vi "Pockels Cal-Interpolate or Condense.vi"(9 "Processing Type (Interpolate)":T1, 11 "Pockels Cal table":string[][](array[string])=[["0", "0", "0", "0"], ["0.1", "", "", ""], ["0.2", "", "6.86", ""], ["0.3", "", "", ""], ["0.4", "37.1", "25.97", "37.1"], ["0.5", "", "", ""], ["0.6", "", "54.39", ""], ["0.7", "", "", ""], ["0.8", "125", "87.5", "125"], ["0.9", "", "", ""], ["1", "", "118.3", ""], ["1.1", "", "", ""], ["1.2", "204", "142.8", "204"], ["1.3", "", "", ""], ["1.4", "", "155.4", ""], ["1.5", "", "", ""], ["1.6", "222", "155.4", "222"], ["1.7", "", "", ""], ["1.8", "", "141.4", ""], ["1.9", "", "", ""], ["2", "152", "106.4", "152"]]) -> (3 "Spline-Interpolated":dbl[][](array[numeric]))   [LabVIEW 2017]
uses:
  Typedefs/Pockels cal processing type.ctl
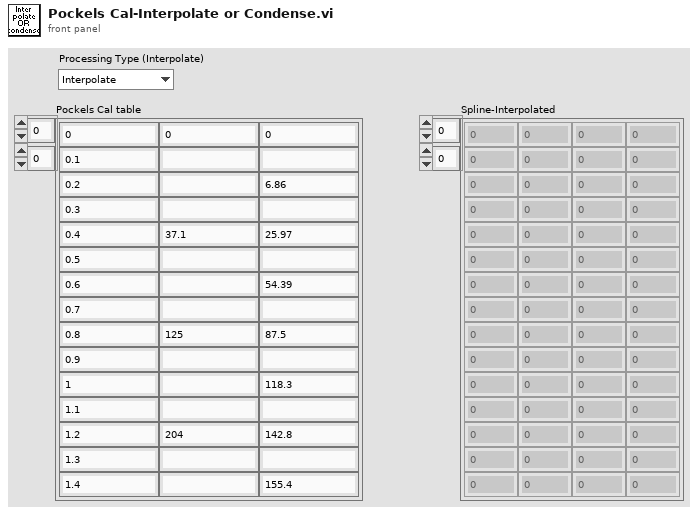
[diagram p1: front panel]
types:
  T1 = typedef "Pockels cal processing type.ctl" = enum16{"Interpolate", "Condense"}
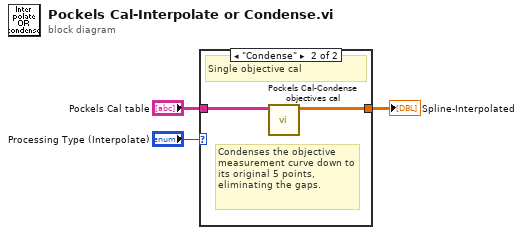
[diagram p0: block diagram]
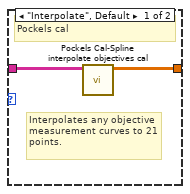
[diagram p2: hidden frame]
diagram:
  n1 = case shown="\"Condense\"" "Processing Type (Interpolate)" {
    tunnel: [w5 w6] -> w3
    tunnel: "Pockels Cal table" -> [w4 w7]
    frame "Interpolate", Default {
      # "Interpolates any objective measurement curves to 21 points."
      # "Pockels cal"
      n2 = call "Pockels Cal-Spline interpolate objectives cal.vi"("Pockels Cal table"=w4) -> ("Spline-Interpolated"=w5:dbl[][])  [unwired: 10 in]
    }
    frame "Condense" {
      # "Condenses the objective measurement curve down to its original 5 points, eliminating the gaps."
      # "Single objective cal"
      n3 = call "Pockels Cal-Condense objectives cal.vi"("Objective power results"=w7) -> ("Condensed objective power results"=w6:dbl[][])  [unwired: 10 in]
    }
  }
  "Spline-Interpolated" <- w3
